vi "Tokenizing Error.vi"(8 "Value Position":i32, 9 "Next Position":i32, 10 "Reason":string, 11 "Tokenizer In":T1) -> (0 "error out":errorcluster, 3 "Tokenizer":T1)   [LabVIEW 2020, in "Stream.lvlib" / "URLPattern.lvclass"]
uses:
  URLPattern.lvclass
  Token Type.ctl
  Token.ctl
  Tokenize Policy.ctl
  Tokenizer.ctl
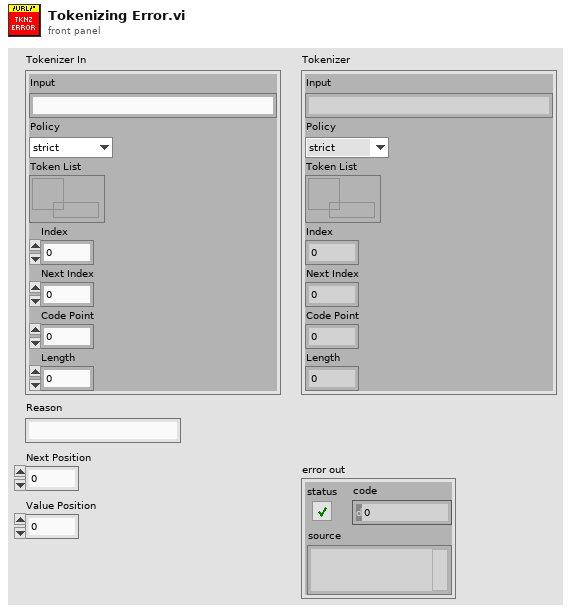
[diagram p1: front panel]
types:
  T1 = typedef "Stream.lvlib/URLPattern.lvclass/Tokenizer.ctl" = cluster{"Input":string, "Policy":T2, "Token List":refnum<queue>, "Index":i32, "Next Index":i32, "Code Point":u32, "Length":i32}
  T2 = typedef "Stream.lvlib/URLPattern.lvclass/Tokenize Policy.ctl" = enum16{"strict", "lenient"}
  T3 = typedef "Stream.lvlib/URLPattern.lvclass/Token Type.ctl" = enum16{"invalid-char", "open", "close", "regexp", "name", "char", "escaped-char", "other-modifier", "asterisk", "end"}
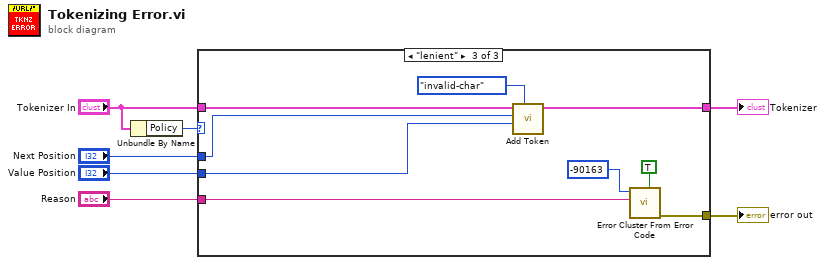
[diagram p0: block diagram]
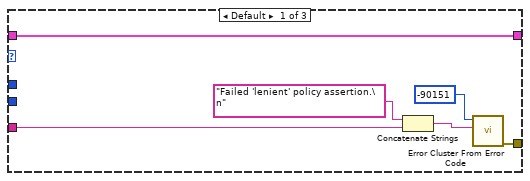
[diagram p2: hidden frame]
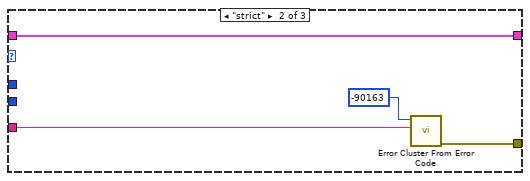
[diagram p3: hidden frame]
diagram:
  n1 = Unbundle By Name("Tokenizer In") -> ("Policy"=w7:T2)
  n2 = case shown="\"lenient\"" w7 {
    tunnel: "Tokenizer In" -> [w9 w15 w26]
    tunnel: [w13 w16 w20] -> w4
    tunnel: [w9 w15 w25] -> w5
    tunnel: "Reason" -> [w8 w14 w18]
    tunnel: "Next Position" -> [_ _ w23]
    tunnel: "Value Position" -> [_ _ w22]
    frame Default {
      n3 = Concatenate Strings("Failed 'lenient' policy assertion.\n" ("string"), w8) -> (w10:string)
      n4 = call <vilib>:"Error Cluster From Error Code.vi"("error message (\"\")"=w10, "error code (0)"=-90151) -> ("error out"=w13:errorcluster)  [unwired: 7 in]
    }
    frame "strict" {
      n5 = call <vilib>:"Error Cluster From Error Code.vi"("error message (\"\")"=w14, "error code (0)"=-90163) -> ("error out"=w16:errorcluster)  [unwired: 7 in]
    }
    frame "lenient" {
      n6 = call "Add Token.vi"("Token Type"=Token_Type."invalid-char", "Value Position"=w22, "Next Position"=w23, "Tokenizer In"=w26) -> ("Tokenizer"=w25:T1)  [unwired: 7 in]
      n7 = call <vilib>:"Error Cluster From Error Code.vi"("is warning? (False)"=TRUE, "error message (\"\")"=w18, "error code (0)"=-90163) -> ("error out"=w20:errorcluster)  [unwired: 6 in]
    }
  }
  "Tokenizer" <- w5
  "error out" <- w4
